vi "Create Container.vi"(8 "Error In":errorcluster, 11 "Splitter Builder in":refnum<class "Splitter Builder.lvclass">) -> (0 "Error Out":errorcluster, 2 "Container":refnum<class "QWidget.lvclass">, 3 "Splitter Builder out":refnum<class "Splitter Builder.lvclass">)   [LabVIEW 2014, in "Splitter Builder.lvclass"]
doc: "Implements the interface provided by Abstract Widget Builder.\n\n\nCopyright (c) 2019 Sze Howe Koh.\nThis code is licensed under the MIT license."
uses:
  Splitter Builder.lvclass
  <vilib>/addons/LQ/Qt Widgets/QWidget/QWidget.lvclass
  Splitter Builder.lvclass/Splitter Builder.ctl
  <vilib>/addons/LQ/Qt Widgets/QSplitter/QSplitter.lvclass
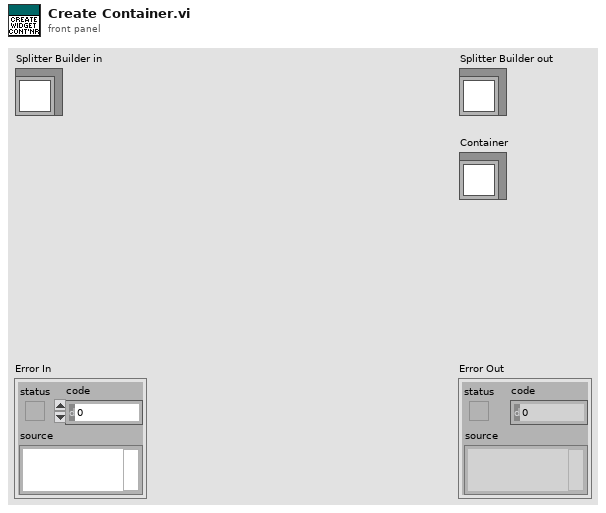
[diagram p1: front panel]
types:
  T1 = typedef "Qt.lvlib/Orientation.ctl" = i32
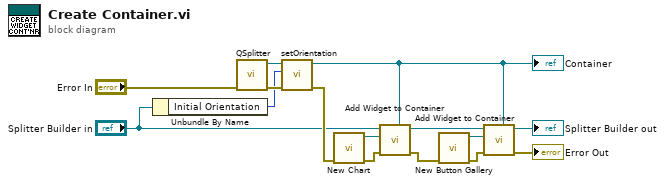
[diagram p0: block diagram]
diagram:
  n1 = Unbundle By Name("Splitter Builder in") -> ("Initial Orientation"=w1:T1)
  n2 = call <vilib>:"QSplitter.vi"("Error In"="Error In") -> ("Error Out"=w4:errorcluster, "New QSplitter"=w6:refnum<class "QSplitter.lvclass">)  [unwired: 9 in]
  n3 = call <vilib>:"setOrientation.vi"("Error In"=w4, "orientation"=w1, "QSplitter In"=w6) -> ("Error Out"=w3:errorcluster, "QSplitter Out"=w5:refnum<class "QSplitter.lvclass">)  [unwired: 7 in]
  "Container" <- w5
  n4 = call "New Chart.vi"("Error In"=w3) -> ("Error Out"=w11:errorcluster, "New LQChart"=w12:refnum<class "LQChart.lvclass">)  [unwired: 9 in]
  n5 = call-dynamic "Add Widget to Container.vi"("Container"=w5, "Error In"=w11, "Widget"=w12, "Splitter Builder in"="Splitter Builder in") -> ("Error Out"=w10:errorcluster, "Splitter Builder out"=w14:refnum<class "Splitter Builder.lvclass">)  [unwired: 6 in]
  n6 = call "New Button Gallery.vi"("Error In"=w10) -> ("Error Out"=w9:errorcluster, "New Button Gallery"=w8:refnum<class "QWidget.lvclass">)  [unwired: 9 in]
  n7 = call-dynamic "Add Widget to Container.vi"("Container"=w5, "Error In"=w9, "Widget"=w8, "Splitter Builder in"=w14) -> ("Error Out"=→"Error Out":errorcluster, "Splitter Builder out"=→"Splitter Builder out":refnum<class "Splitter Builder.lvclass">)  [unwired: 6 in]
